vi "ALTS-2015 Check for Clamp Status .vi"(8 "error in (no error)":errorcluster, 11 "Station Cluster":T1) -> (0 "error out":errorcluster, 3 "Clamp?":bool)   [LabVIEW 2013]
doc: "Copyright © 2005, Soliton Technologies.\nAll rights reserved."
uses:
  Controls/ALTS-2015 Station Cluster.ctl
  SLL DAQ Engine/Software/Source Code/Sub VIs/DAQ Engine/Controls/SLL DE DI Global Options.ctl
  SLL DAQ Engine/Software/Source Code/Sub VIs/DAQ Engine/Controls/SLL DE List of Digital Inputs.ctl
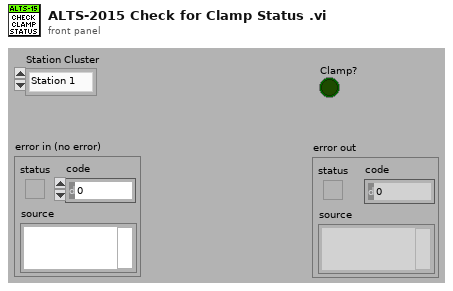
[diagram p1: front panel]
types:
  T1 = typedef "ALTS-2015 Station Cluster.ctl" = enum16{"Station 1", "Station 2", "Station 3", "Station 4"}
  T2 = typedef "SLL DE DI Global Options.ctl" = enum16{"Init", "Write Line", "Write Array", "Read Line", "Read Array", "Read Full Status", "Write Full Status"}
  T3 = typedef "SLL DE List of Digital Inputs.ctl" = enum16{"STATION1_START", "STATION1_STOP", "STATION1_CLAMPED", "STATION1_TC_PASS", "STATION1_TC_FAIL", "STATION1_TTA", "STATION1_TTB", "STATION2_START", "STATION2_STOP", "STATION2_CLAMPED", "STATION2_TC_PASS", "STATION2_TC_FAIL", "STATION2_TTA", "STATION2_TTB", "STATION3_START", "STATION3_STOP", "STATION3_CLAMPED", "STATION3_TC_PASS", "STATION3_TC_FAIL", "STATION3_TTA", "STATION3_TTB", "STATION4_START", "STATION4_STOP", "STATION4_CLAMPED", "STATION4_TC_PASS", "STATION4_TC_FAIL", "STATION4_TTA", "STATION4_TTB"}
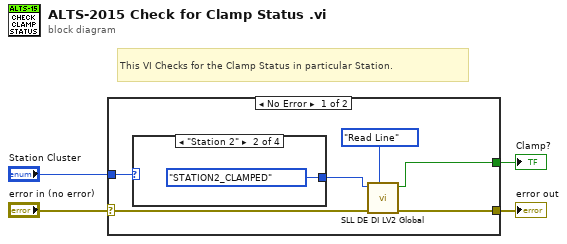
[diagram p0: block diagram]
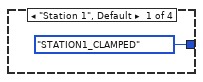
[diagram p2: hidden frame]
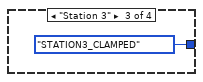
[diagram p3: hidden frame]
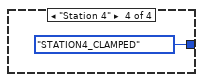
[diagram p4: hidden frame]
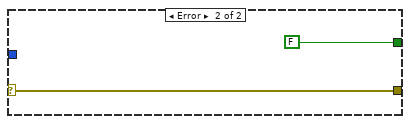
[diagram p5: hidden frame]
diagram:
  # "This VI Checks for the Clamp Status in particular Station."
  n1 = case shown="No Error" "error in (no error)" {
    selector: "error in (no error)" -> [w7 w16]
    tunnel: [w6 w16] -> w3
    tunnel: [w8 FALSE ("Digital Line Status")] -> w1
    tunnel: "Station Cluster" -> [w5 _]
    frame No Error {
      n2 = case shown="\"Station 2\"" w5 {
        tunnel: [SLL_DE_List_of_Digital_Inputs."STATION1_CLAMPED" ("DI Channel Name") SLL_DE_List_of_Digital_Inputs."STATION2_CLAMPED" ("DI Channel Name") SLL_DE_List_of_Digital_Inputs."STATION3_CLAMPED" ("DI Channel Name") SLL_DE_List_of_Digital_Inputs."STATION4_CLAMPED" ("DI Channel Name")] -> w9
        frame "Station 1", Default {
        }
        frame "Station 2" {
        }
        frame "Station 3" {
        }
        frame "Station 4" {
        }
      }
      n3 = call "SLL DE DI LV2 Global.vi"("Option"=SLL_DE_DI_Global_Options."Read Line", "error in (no error)"=w7, "DI Channel Name"=w9) -> ("error out"=w6:errorcluster, "Digital Line Status"=w8:bool)  [unwired: 5 in, 2 out]
    }
    frame Error {
    }
  }
  "error out" <- w3
  "Clamp?" <- w1
